vi "VI_PowerSpectrum.v1.0.vi"() -> ()   [LabVIEW 2018]
uses:
  <vilib>/Analysis/2dsp.llb/Real FFT.vi
  <vilib>/measure/maspectr.llb/FFT Power Spectrum and PSD for 1 Chan.vi
  <vilib>/rtlsdr/rtlsdr.lvlib
  <vilib>/measure/NI_MAPro.lvlib
  <vilib>/Analysis/NI_AALPro.lvlib
panel:
  out "Power Spectrum FFt":dbl[](graph)
  out "Power Spectrum":cluster{"f0":dbl, "df":dbl, "magnitude":dbl[]}(graph)
  out "Center Frequency":dbl
  in  "config":bool
  in  "Number Of Samples":i32
  in  "Center Frequency":u32
  in  "Sample Rate":u32
  out "function return":i32
  in  "Device Index":u32
  out "Device USB Strings":T1
  out "DeviceRefnum Out":u64
  in  "stop":bool
  out "Device Count":u32
  # "1"
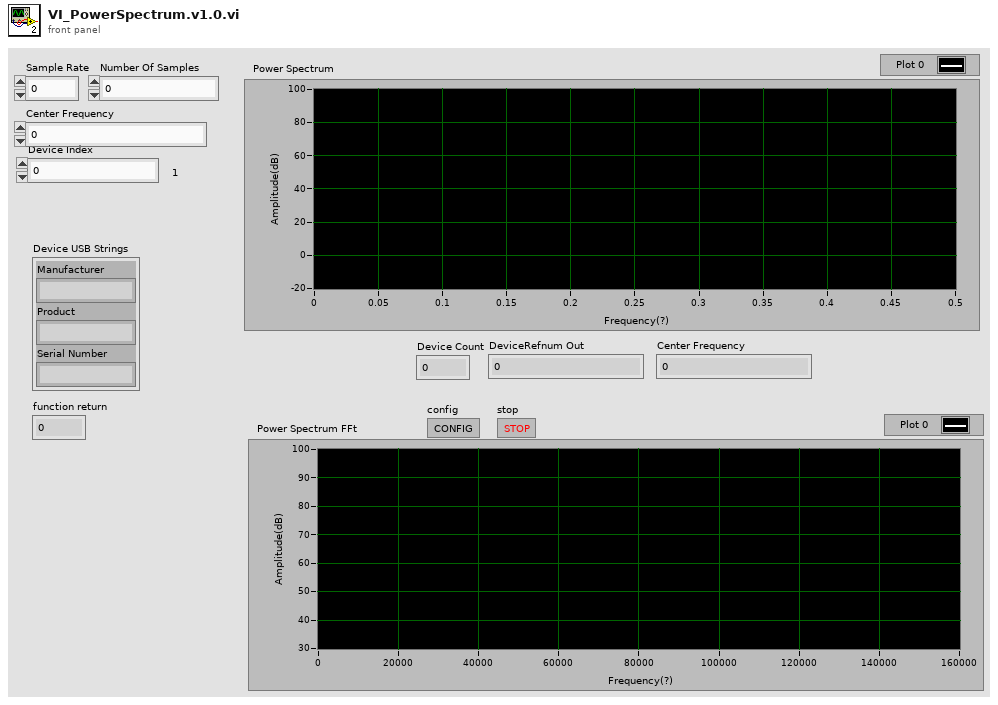
[diagram p1: front panel]
types:
  T1 = cluster{"Manufacturer":string, "Product":string, "Serial Number":string}
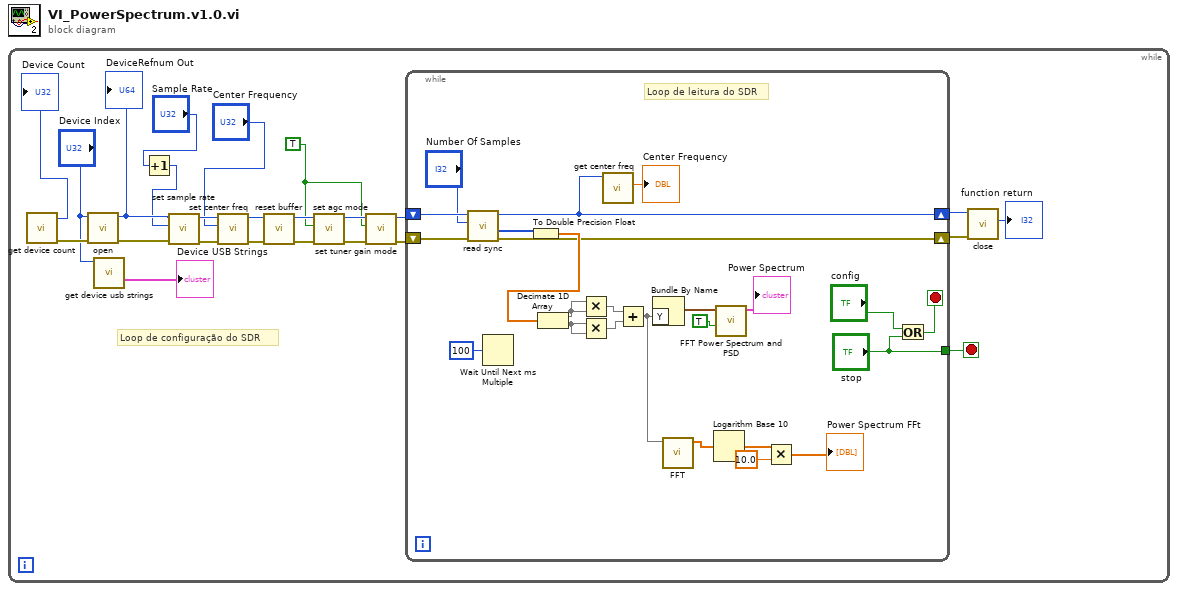
[diagram p0: block diagram]
diagram:
  n1 = while {
    stop <- w3 stop-if-true
    w8 = TRUE ("AGC Enable")
    # "Loop de configuração do SDR"
    n2 = call <vilib>:"get device count.vi"() -> ("error out"=w23:errorcluster, "Device Count"=→"Device Count":u32)  [unwired: 10 in]
    n3 = call <vilib>:"open.vi"("error in (no error)"=w23, "Device Index"="Device Index") -> ("error out"=w19:errorcluster, "DeviceRefnum Out"=w18:u64)  [unwired: 6 in]
    "DeviceRefnum Out" <- w18
    n4 = call <vilib>:"get device usb strings.vi"("Device Index"="Device Index") -> ("Device USB Strings"=→"Device USB Strings":T1)  [unwired: 8 in, 2 out]
    n5 = Increment(x="Sample Rate") -> (x+1=w1:u32)
    n6 = call <vilib>:"set sample rate.vi"("error in (no error)"=w19, "Sample Rate"=w1, "DeviceRefnum"=w18) -> ("error out"=w17:errorcluster, "DeviceRefnum Out"=w16:u64)  [unwired: 6 in, 1 out]
    n7 = call <vilib>:"set center freq.vi"("error in (no error)"=w17, "Center Frequency"="Center Frequency", "DeviceRefnum"=w16) -> ("error out"=w15:errorcluster, "DeviceRefnum Out"=w14:u64)  [unwired: 6 in, 1 out]
    n8 = call <vilib>:"reset buffer.vi"("error in (no error)"=w15, "DeviceRefnum"=w14) -> ("error out"=w12:errorcluster, "DeviceRefnum Out"=w11:u64)  [unwired: 7 in, 1 out]
    n9 = call <vilib>:"set agc mode.vi"("error in (no error)"=w12, "AGC Enable"=w8, "DeviceRefnum"=w11) -> ("error out"=w10:errorcluster, "DeviceRefnum Out"=w9:u64)  [unwired: 6 in, 1 out]
    n10 = call <vilib>:"set tuner gain mode.vi"("error in (no error)"=w10, "AutoGain"=w8, "DeviceRefnum"=w9) -> ("error out"=w7:errorcluster, "DeviceRefnum Out"=w6:u64)  [unwired: 6 in, 1 out]
    n11 = while {
      shift-right: [w38] -> w4
      shift-left: w6 -> [w47]
      shift-right: [w43] -> w5
      shift-left: w7 -> [w48]
      tunnel: ["stop"] -> w3
      stop <- w41 stop-if-true
      # "Loop de leitura do SDR"
      n12 = call <vilib>:"read sync.vi"("error in (no error)"=w48, "Number Of Samples"="Number Of Samples", "DeviceRefnum"=w47) -> ("error out"=w43:errorcluster, "Sample Buffer"=w44:u8[], "DeviceRefnum Out"=w38:u64)  [unwired: 5 in, 1 out]
      n13 = Wait Until Next ms Multiple(millisecond multiple=u32 100) -> ()  [unwired: 1 out]
      n14 = To Double Precision Float(number=w44) -> (double precision float=w45:dbl[])
      n15 = Decimate 1D Array(w45) -> (w36:dbl[], w35:dbl[])
      n16 = Multiply(x=w36, y=w36) -> (x*y=w34:dbl[])
      n17 = Multiply(x=w35, y=w35) -> (x*y=w33:dbl[])
      n18 = call <vilib>:"get center freq.vi"("DeviceRefnum"=w38) -> ("Center Frequency"=→"Center Frequency":dbl)  [unwired: 8 in, 2 out]
      n19 = Add(x=w34, y=w33) -> (x+y=w29:dbl[])
      n20 = Bundle By Name("Y"=w29) -> (w32:waveform(dbl))  [unwired: 1 in]
      n21 = call-poly <vilib>:"FFT.vi"("X"=w29) -> ("FFT {X}"=w28:cdb[])  [unwired: 9 in, 1 out]
      n22 = Logarithm Base 10(1:w28) -> (0:w26:cdb[])
      n23 = call-poly <vilib>:"FFT Power Spectrum and PSD.vi"("dB On (F)"=TRUE, "time signal"=w32) -> ("Power Spectrum / PSD"=→"Power Spectrum":cluster{"f0":dbl, "df":dbl, "magnitude":dbl[]})  [unwired: 6 in, 3 out]
      n24 = Multiply(x=w26, y=10.0) -> (x*y=→"Power Spectrum FFt":cdb[])
      n25 = Or(x="config", y="stop") -> (x .or. y?=w41:bool)
    }
    n26 = call <vilib>:"close.vi"("error in (no error)"=w5, "DeviceRefnum"=w4) -> ("function return"=→"function return":i32)  [unwired: 8 in, 1 out]
  }
